vi "Car_Speed_R92A.vi"(10 "精度":dbl=1.0, 11 "车速":u16) -> (3 "报文":T1 {"[7]" format="%02x"; "[6]" format="%02x"; "[5]" format="%02x"; "[4]" format="%02x"; "[3]" format="%02x"; "[2]" format="%02x"; "[1]" format="%02x"; "[0]" format="%02x"})   [LabVIEW 2020]
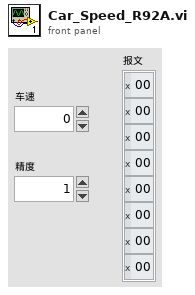
[diagram p1: front panel]
types:
  T1 = cluster{"[0]":u8, "[1]":u8, "[2]":u8, "[3]":u8, "[4]":u8, "[5]":u8, "[6]":u8, "[7]":u8}
  T2 = cluster{u8, u8, "y":u8, "y":u8, "y":u8, "y":u8, "y":u8, "y":u8}
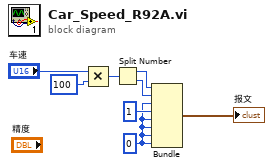
[diagram p0: block diagram]
diagram:
  w3 = u8 0 ("y")
  n1 = Multiply(x="车速", y=u16 100) -> (x*y=w7:u16)
  n2 = Split Number(x=w7) -> (hi(x)=w6:u8, lo(x)=w5:u8)
  n3 = Bundle(w6, w5, "y"=w3, "y"=u8 1, "y"=w3, "y"=w3, "y"=w3, "y"=w3) -> (→"报文":T2)  [unwired: 1 in]
